vi "Pop Up.vi"(11 "Ex Queue Actor in":refnum<class "Ex Queue Actor.lvclass">) -> (3 "Ex Queue Actor out":refnum<class "Ex Queue Actor.lvclass">)   [LabVIEW 2021, in "Ex Queue Actor.lvlib" / "Ex Queue Actor.lvclass"]
uses:
  Ex Queue Actor.lvclass
  Ex Queue Actor.lvclass/Ex Queue Actor.ctl
  Actor/Msgs/Create/Create Msg/Create Msg.lvclass
  C:/git/jettl/src/Actor/Actor/Actor.lvclass
  C:/git/jettl/src/Actor/Msgs/Teardown/Teardown/Teardown.lvclass
  C:/git/jettl/src/Actor/Queue Actor/Queue Actor.lvclass
  C:/git/jettl/src/Actor/Msgs/Create/Create/Create.lvclass
  C:/git/jettl/src/Actor/Msgs/Event Last Ack/Event Last Ack/Event Last Ack.lvclass
  C:/git/jettl/src/Actor/Msgs/Queue Last Ack/Queue Last Ack/Queue Last Ack.lvclass
  C:/git/jettl/src/Example/Ex Queue Actor/Ex Queue Actor/Ex Queue Actor.lvclass
  C:/git/jettl/src/Example/Pop Up/Pop Up/Pop Up.lvclass
  C:/git/jettl/src/Actor/Msgs/Create/Create Msg/Create Msg.lvclass
  C:/git/jettl/src/Actor/Msg/Msg.lvclass
  <vilib>/numeric/Random Number (Range) U64.vi
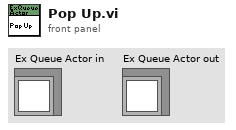
[diagram p1: front panel]
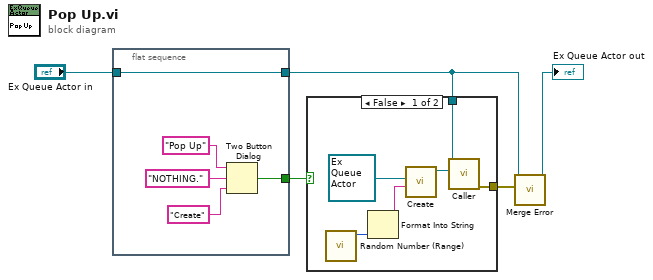
[diagram p0: block diagram]
diagram:
  n1 = flat-sequence {
    tunnel: [w10] -> w1
    tunnel: "Ex Queue Actor in" -> [w10]
    tunnel: [w7] -> w4
    frame #0 {
      n2 = Two Button Dialog(message="Pop Up", 1:"Create" ("F button name (\"Cancel\")"), 2:"NOTHING." ("T button name (\"OK\")")) -> (T button?=w7:bool)
    }
  }
  n3 = case shown="False" w4 {
    tunnel: w1 -> [w12 _]
    tunnel: [w11 _] -> w2
    frame False {
      n4 = call-poly <vilib>:"Random Number (Range).vi"() -> ("number"=w15:u64)  [unwired: 11 in]
      n5 = Format Into String(w15) -> (resulting string=w14:string)  [unwired: 3 in, 1 out]
      n6 = call "Create.vi"("Alias"=w14, "Actor"=refnum<class "Ex Queue Actor.lvclass"> refnum ("Dev Actor.lvlib:Dev Actor.lvclass")) -> ("Create Msg out"=w13:refnum<class "Create Msg.lvclass">)  [unwired: 9 in]
      n7 = call-dynamic "Caller.vi"("Msg"=w13, "Ex Queue Actor in"=w12) -> ("error out"=w11:errorcluster)  [unwired: 9 in]
    }
    frame True {
    }
  }
  n8 = call-dynamic "Merge Error.vi"("Error"=w2, "Ex Queue Actor in"=w1) -> ("Ex Queue Actor out"=→"Ex Queue Actor out":refnum<class "Ex Queue Actor.lvclass">)  [unwired: 9 in]
